vi "write_to_file.vi"(0 "refnum":refnum<file>, 1 "Time":dbl, 5 "y data":dbl, 7 "y data precision":i16, 9 "x data":dbl, 11 "x data precision":i16, 12 "Setpoint":dbl) -> (4 "dup refnum":refnum<file>)   [LabVIEW 2012]
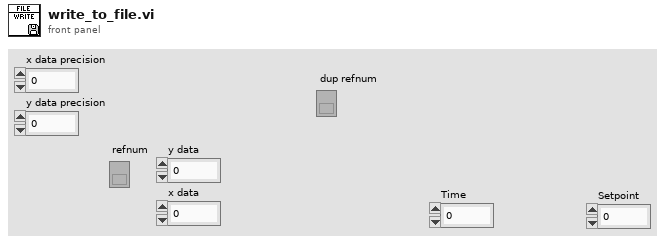
[diagram p1: front panel]
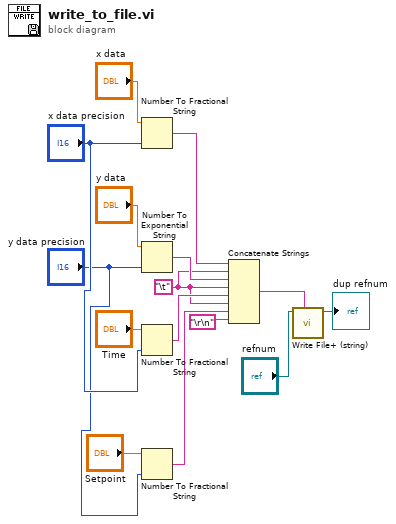
[diagram p0: block diagram]
diagram:
  w6 = "\t"
  n1 = Number To Fractional String(number="x data", precision (6)="x data precision") -> (F-format string=w14:string)  [unwired: 2 in]
  n2 = Number To Exponential String(number="y data", precision (6)="y data precision") -> (E-format string=w13:string)  [unwired: 2 in]
  n3 = Number To Fractional String(number="Time", precision (6)="x data precision") -> (F-format string=w7:string)  [unwired: 2 in]
  n4 = Number To Fractional String(number="Setpoint", precision (6)="y data precision") -> (F-format string=w5:string)  [unwired: 2 in]
  n5 = Concatenate Strings(w14, w6, w13, w6, w7, w6, w5, "\r\n") -> (w15:string)
  n6 = call <vilib>:"Write File+ (string).vi"("string"=w15, "refnum"="refnum") -> ("dup refnum"=→"dup refnum":refnum<file>)  [unwired: 5 in, 2 out]
